vi "Host_NetStreams.vi"   [LabVIEW 2019]
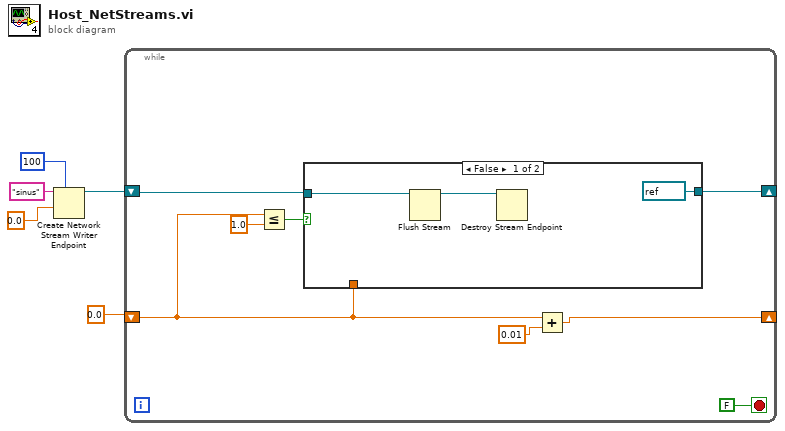
[diagram p0: block diagram]
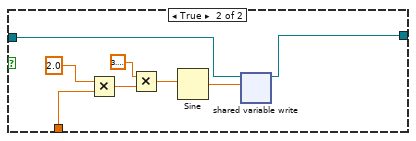
[diagram p2: hidden frame]
diagram:
  n1 = Create Network Stream Writer Endpoint(7:100 ("writer buffer size"), 9:0.0 ("y"), 11:"sinus" ("writer name")) -> (3:w4:refnum<k21>)  [unwired: 4 in, 1 out]
  n2 = while {
    shift-right: [w12] -> _
    shift-left: 0.0 -> [w9]
    shift-right: [w6] -> _
    shift-left: w4 -> [w7]
    stop <- FALSE stop-if-true
    n3 = Less Or Equal?(x=w9, y=1.0) -> (x <= y?=w10:bool)
    n4 = case shown="False" w10 {
      tunnel: w9 -> [_ w20]
      tunnel: w7 -> [w16 w18]
      tunnel: [refnum<k21> refnum ("writer name") w17] -> w6
      frame False {
        n5 = Flush Stream(11:w16) -> (3:w15:refnum<k21>)  [unwired: 3 in, 2 out]
        n6 = Destroy Stream Endpoint(11:w15) -> ()  [unwired: 1 in, 1 out]
      }
      frame True {
        n7 = Multiply(x=2.0 ("x*y"), y=w20) -> (x*y=w23:dbl)
        n8 = Multiply(x=3.141592653589793, y=w23) -> (x*y=w22:dbl)
        n9 = Sine(x=w22) -> (sin(x)=w19:dbl)
        n10 = shared-variable-write(w18, w19) -> (w17:refnum<k21>)  [unwired: 2 in, 2 out]
      }
    }
    n11 = Add(x=w9, y=0.01) -> (x+y=w12:dbl)
  }
